vi "New Node On Wire_CREATE.vi"(8 "error in":errorcluster, 10 "New Node position":cluster{"Left":i32, "Top":i32}, 11 "Wire in":refnum<vi>) -> (0 "error out":errorcluster, 2 "First wired terminal":refnum<vi>, 3 "Temporary Node":refnum<vi>)   [LabVIEW 2023]
doc: "This VI creates a new node on a wire at the position indicated. You can wire any other terminal to the New Node Terminal, and later you will need to destroy the temporary function used to create the new node by using the New Node On Wire_CLEANUP.vi.\n\nThis VI works by placing a subVI with variant inputs and outputs on the wire, wiring the input and output terminals together, and passing our the reference to the source terminal. \n\nReturns first wired terminal (will l be sink if wire was borken). Subsequent placement of new objects are relative to this terminal."
panel:
  out "Array":bool[](array[boolean])
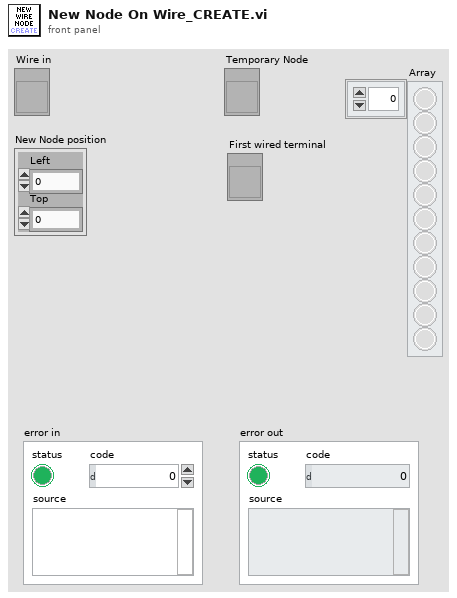
[diagram p1: front panel]
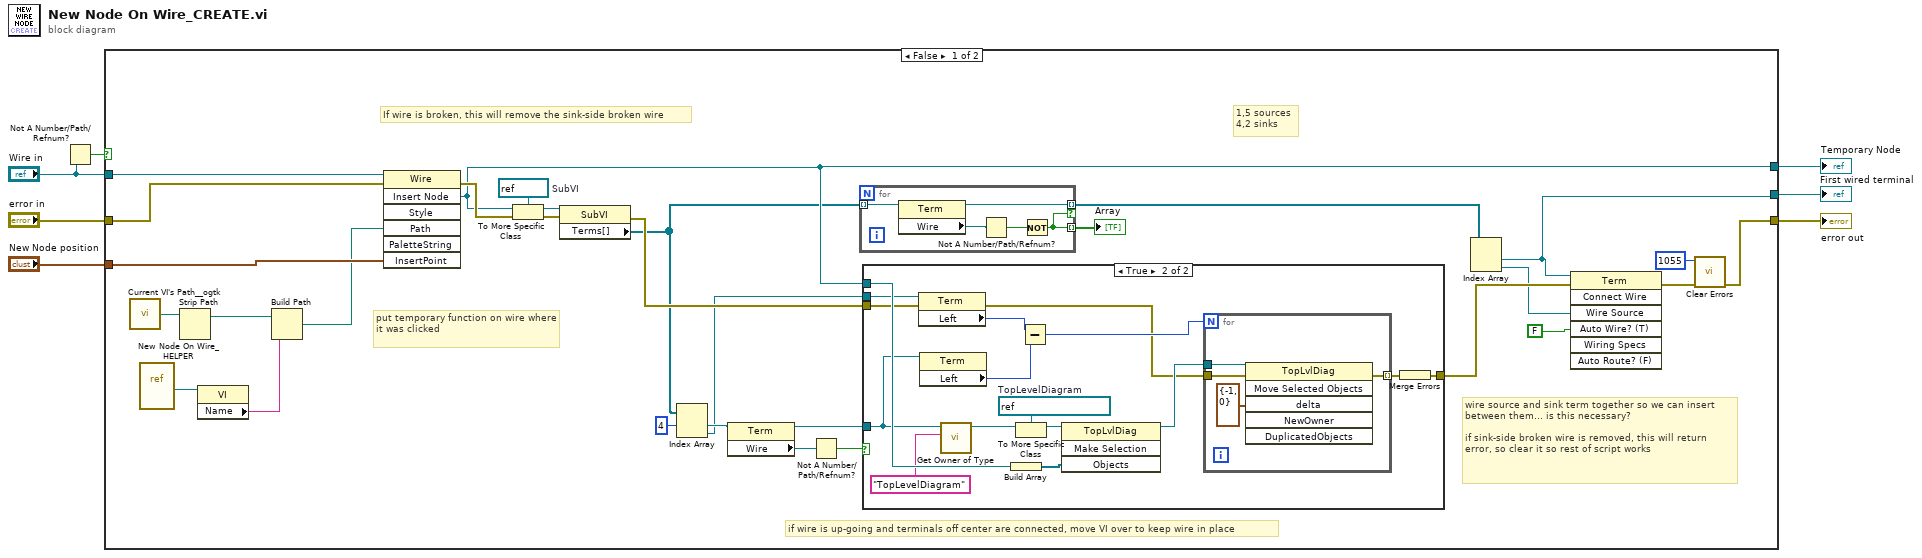
[diagram p0: block diagram]
diagram:
  n1 = Not A Number/Path/Refnum?(number/path/refnum="Wire in") -> (NaN/Path/Refnum?=w1:bool)
  n2 = case shown="False" w1 {
    tunnel: [w27 _] -> w7
    tunnel: "New Node position" -> [w33 _]
    tunnel: [w8 _] -> w5
    tunnel: "error in" -> [w32 w64]
    tunnel: [w10 w64] -> w3
    tunnel: "Wire in" -> [w31 _]
    frame False {
      w35 = refnum<vi> refnum  # SubVI
      # "wire source and sink term together so we can insert between them... is this necessary?\n\nif sink-side broken wire is removed, this will return error, so clear it so rest of script works"
      # "1,5 sources \n4,2 sinks"
      # "If wire is broken, this will remove the sink-side broken wire"
      # "if wire is up-going and terminals off center are connected, move VI over to keep wire in place"
      # "put temporary function on wire where it was clicked"
      n3 = call <userlib>:"Current VI's Path__ogtk.vi"() -> ("Current VI's Path (+ Relative)"=w14:path)  [unwired: 1 in]
      n4 = vi-ref "New Node On Wire_HELPER.vi"() -> (w15:refnum<vi>)
      n5 = Strip Path(path=w14) -> (stripped path=w13:path)  [unwired: 1 out]
      n6 = property class="VI"(reference=w15) -> ("Name"=w12:string)  [unwired: 1 in, 2 out]
      n7 = Build Path(base path=w13, name or relative path=w12) -> (appended path=w11:path)
      n8 = invoke class="Wire" method="Insert Node"(reference=w31, error in=w32, "Path"=w11, "InsertPoint"=w33) -> (error out=w36:errorcluster, "Insert Node"=w27:refnum<vi>)  [unwired: 3 in, 5 out]
      n9 = To More Specific Class(target class=w35, reference=w27, error in=w36) -> (specific class reference=w34:refnum<vi>, error out=w37:errorcluster)
      n10 = property class="SubVI"(reference=w34, error in=w37) -> (error out=w24:errorcluster, "Terms[]"=w20:refnum<vi>[])  [unwired: 1 out]
      n11 = Index Array(array=w20, index #1=4 ("index")) -> (element #1=w22:refnum<vi>, element #2=w21:refnum<vi>)  [unwired: 1 in]
      n12 = property class="Term"(reference=w22) -> (reference out=w28:refnum<vi>, "Wire"=w30:refnum<vi>)  [unwired: 1 in, 1 out]
      n13 = Not A Number/Path/Refnum?(number/path/refnum=w30) -> (NaN/Path/Refnum?=w29:bool)
      n14 = for {
        tunnel: w20 -> [w42] mode=indexing
        tunnel: [w38] -> w19 mode=indexing
        tunnel: [w39] -> w18 mode=indexing if=w38
        n15 = property class="Term"(reference=w42) -> (reference out=w39:refnum<vi>, "Wire"=w41:refnum<vi>)  [unwired: 1 in, 1 out]
        n16 = Not A Number/Path/Refnum?(number/path/refnum=w41) -> (NaN/Path/Refnum?=w40:bool)
        n17 = Not(x=w40) -> (.not. x?=w38:bool)
      }
      "Array" <- w19
      n18 = case shown="True" w29 {
        tunnel: w28 -> [_ w44]
        tunnel: w27 -> [_ w53]
        tunnel: [w43 w46] -> w25
        tunnel: w24 -> [w43 w48]
        tunnel: w21 -> [_ w45]
        frame False {
        }
        frame True {
          w54 = refnum<vi> refnum  # TopLevelDiagram
          n19 = property class="Term"(reference=w45, error in=w48) -> (error out=w47:errorcluster, "Left"=w59:i32)  [unwired: 1 out]
          n20 = property class="Term"(reference=w44) -> ("Left"=w58:i32)  [unwired: 1 in, 2 out]
          n21 = call "Get Owner of Type.vi"("Owner Class Name desired"="TopLevelDiagram", "reference"=w44) -> ("Owner of Type"=w50:refnum<vi>)  [unwired: 5 in, 4 out]
          n22 = Build Array(w53) -> (w56:refnum<vi>[])
          n23 = To More Specific Class(target class=w54, reference=w50) -> (specific class reference=w55:refnum<vi>)  [unwired: 1 in, 1 out]
          n24 = Subtract(x=w59, y=w58) -> (x-y=w52:i32)
          n25 = invoke class="TopLvlDiag" method="Make Selection"(reference=w55, "Objects"=w56) -> (reference out=w57:refnum<vi>)  [unwired: 2 in, 3 out]
          n26 = for {
            N: w52 -> [_]
            tunnel: w57 -> [w63]
            tunnel: [w61] -> w49 mode=indexing
            tunnel: w47 -> [w60]
            n27 = invoke class="TopLvlDiag" method="Move Selected Objects"(reference=w63, error in=w60, "delta"=cluster{"X":i32, "Y":i32} {"X"=-1, "Y"=0} ("X/Y Delta")) -> (error out=w61:errorcluster)  [unwired: 3 in, 5 out]
          }
          n28 = Merge Errors(w49) -> (w46:errorcluster)
        }
      }
      n29 = Index Array(array=w18) -> (element #1=w8:refnum<vi>, element #2=w16:refnum<vi>)  [unwired: 2 in]
      n30 = invoke class="Term" method="Connect Wire"(reference=w8, error in=w25, "Wire Source"=w16, "Auto Wire? (T)"=FALSE) -> (error out=w17:errorcluster)  [unwired: 3 in, 6 out]
      n31 = call <vilib>:"Clear Errors.vi"("error in (no error)"=w17, "specific error code to clear (0: all)"=1055) -> ("error out"=w10:errorcluster)  [unwired: 4 in, 1 out]
    }
    frame True {
    }
  }
  "Temporary Node" <- w7
  "First wired terminal" <- w5
  "error out" <- w3
